vi "Fan Speed Initialization.vi"(8 "error in":errorcluster) -> (0 "error out":errorcluster, 3 "DAQmx Task Out":refnum<k21>)   [LabVIEW 2020]
uses:
  <vilib>/DAQmx/create/channels.llb/DAQmx Create Channel (CI-Frequency).vi
  <vilib>/DAQmx/configure/timing.llb/DAQmx Timing (Implicit).vi
  <resource>/objmgr/daqmx.rc
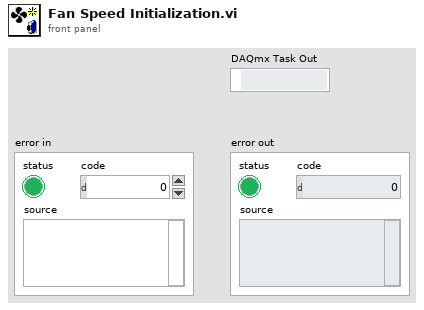
[diagram p1: front panel]
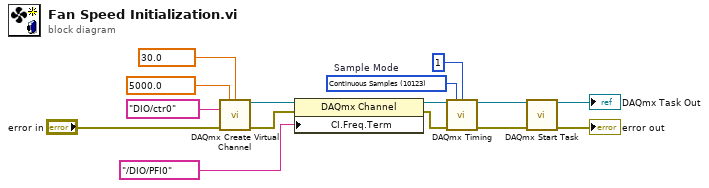
[diagram p0: block diagram]
diagram:
  w15 = 10123 items=["Finite Samples"=10178, "Continuous Samples"=10123, "Hardware Timed Single Point"=12522]  # Sample Mode
  n1 = call-poly <vilib>:"DAQmx Create Virtual Channel.vi"("maximum value"=5000.0 ("Max Frequency"), "minimum value"=30.0 ("Min Frequency"), "counter"=tag "DIO/ctr0" ("Counter"), "error in"="error in") -> ("task out"=w12:refnum<k21>, "error out"=w11:errorcluster)  [unwired: 10 in]
  n2 = property class="DAQmx Channel"(reference=w12, error in=w11, "CI.Freq.Term"=tag "/DIO/PFI0" ("Frequency Input Terminal")) -> (reference out=w13:refnum<k21>, error out=w14:errorcluster)
  n3 = call-poly <vilib>:"DAQmx Timing.vi"("task/channels in"=w13, "sample mode"=w15, "samples per channel"=1, "error in"=w14) -> ("task out"=w7:refnum<k21>, "error out"=w6:errorcluster)  [unwired: 10 in]
  n4 = call <vilib>:"DAQmx Start Task.vi"("task/channels in"=w7, "error in"=w6) -> ("task out"=→"DAQmx Task Out":refnum<k21>, "error out"=→"error out":errorcluster)  [unwired: 12 in]
